vi "Actor Core.vi"(8 "error in":errorcluster, 11 "Nested in":refnum<class "Measurement GEN.lvclass">) -> (0 "error out":errorcluster, 3 "Actor out":refnum<class "Actor.lvclass">)   [LabVIEW 2020, in "Measurement GEN.lvlib" / "Measurement GEN.lvclass"]
doc: "(<B>Filename</B>: Actor Framework.lvlib:Actor.lvclass:Actor Core.vi)\n\nReceives messages to the actor, reacts to them, and initiates any error handling that may shut the actor down.\n\nDescendant classes may override this VI to append parallel tasks for the actor to complete while it handles messages. Overrides use the Call Parent Method node."
uses:
  Measurement GEN.lvclass
  <vilib>/ActorFramework/Stop Msg/Stop Msg.lvclass
  <vilib>/ActorFramework/Actor/Actor.lvclass
  F Generator Messages/Graficar datos Msg/Graficar datos Msg.lvclass
  <vilib>/measure/NI_MABase.lvlib
  C:/Program Files/National Instruments/LabVIEW 2020/vi.lib/ActorFramework/Actor/Actor.lvclass
  C:/Users/deLili/Desktop/UDLSB IET/701/Instrumentacion Virtual/Fork/AF-CML-TAREA/AF-CML-Tarea/Measurement GEN/Measurement GEN.lvclass
types:
  T1 = cluster{"Frecuencia":refnum<user-event>, "Amplitud":refnum<user-event>, "Stop":refnum<user-event>, "Start/Stop HL":refnum<user-event>, "Tipo Señal":refnum<user-event>}
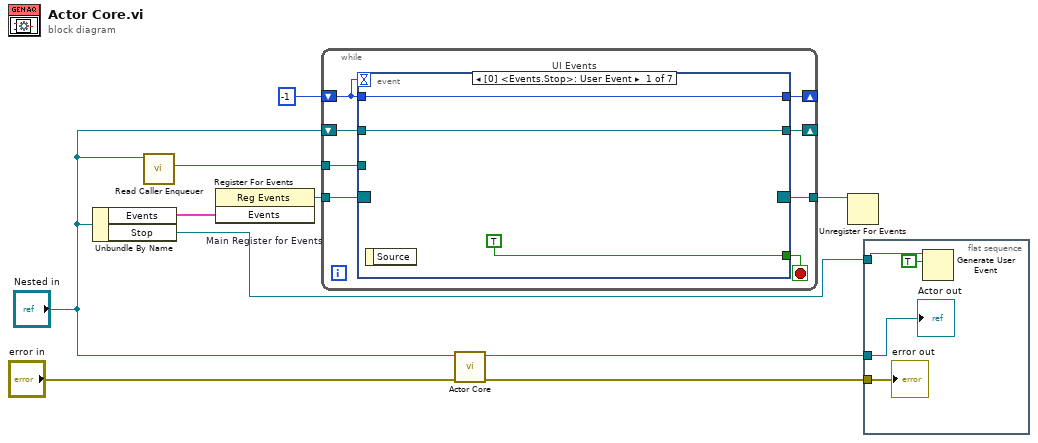
[diagram p0: block diagram]
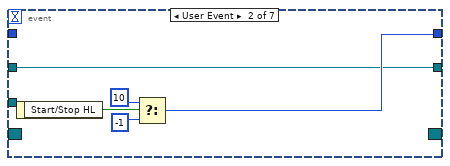
[diagram p2: hidden frame]
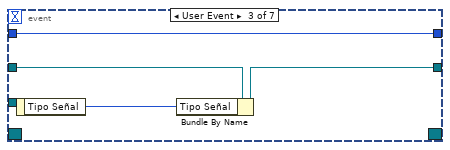
[diagram p3: hidden frame]
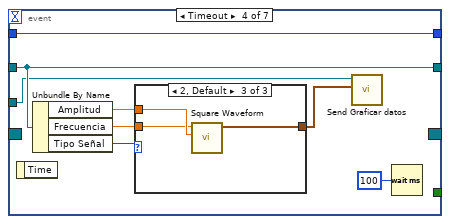
[diagram p4: hidden frame]
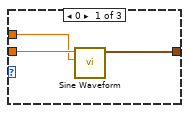
[diagram p5: hidden frame]
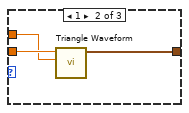
[diagram p6: hidden frame]
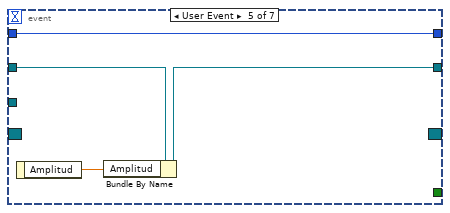
[diagram p7: hidden frame]
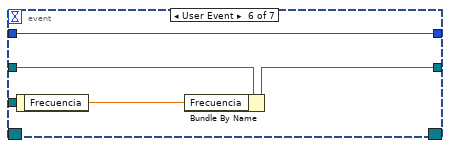
[diagram p8: hidden frame]
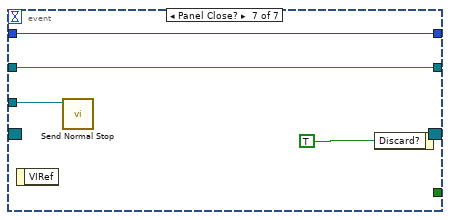
[diagram p9: hidden frame]
diagram:
  n1 = Unbundle By Name("Nested in") -> ("Events"=w7:T1, "Stop"=w4:refnum<user-event>)
  n2 = call <vilib>:"Read Caller Enqueuer.vi"("Actor"="Nested in") -> ("Caller Enqueuer"=w1:refnum<class "Message Enqueuer.lvclass">)  [unwired: 10 in]
  n3 = register-events "Main Register for Events"(w7) -> (reference out=w8:refnum<event-registration>)  [unwired: 2 in, 1 out]
  n4 = while {
    tunnel: w8 -> [w11]
    tunnel: [w17] -> w6
    shift-right: [w14] -> _
    shift-left: -1 -> [w15]
    shift-right: [w13] -> _
    shift-left: "Nested in" -> [w16]
    tunnel: w1 -> [w12]
    stop <- w18 stop-if-true
    n5 = event "UI Events" shown="[0] <Events.Stop>: User Event" {
      selector: w11 -> [_ _ _ _ _ _ _]
      dyn-events: [_ _ _ _ _ _ _] -> w17
      timeout: w15 -> [_ _ _ _ _ _ _]
      tunnel: [TRUE _ _ _ _ _ _] -> w18
      tunnel: w16 -> [w20 w22 w29 w37 w50 w55 w57]
      tunnel: w15 -> [w19 _ w30 w38 w51 w54 w58]
      tunnel: [w19 w23 w30 w38 w51 w54 w58] -> w14
      tunnel: [w20 w22 w28 w37 w49 w53 w57] -> w13
      tunnel: w12 -> [_ _ _ w36 _ _ w56]
      event User Event {
        n6 = event-data() -> ()  [unwired: 1 in, 1 out]
      }
      event User Event {
        n7 = event-data() -> ("Start/Stop HL"=w26:bool)  [unwired: 1 in]
        n8 = Select(t=10, s=w26, f=-1) -> (s? t:f=w23:i32)
      }
      event User Event {
        n9 = event-data() -> ("Tipo Señal"=w27:u16)  [unwired: 1 in]
        n10 = Bundle By Name(cluster=w29, "Tipo Señal"=w27) -> (w28:refnum<class "Measurement GEN.lvclass">)
      }
      event Timeout {
        n11 = event-data() -> ()  [unwired: 1 in, 1 out]
        n12 = Unbundle By Name(w37) -> ("Amplitud"=w32:dbl, "Frecuencia"=w33:dbl, "Tipo Señal"=w34:u16)
        n13 = case shown="2, Default" w34 {
          tunnel: w33 -> [w41 w44 w46]
          tunnel: w32 -> [w40 w43 w47]
          tunnel: [w39 w42 w45] -> w31
          frame 0 {
            n14 = call <vilib>:"Sine Waveform.vi"("amplitude"=w40, "frequency"=w41) -> ("signal out"=w39:waveform(dbl))  [unwired: 8 in, 1 out]
          }
          frame 1 {
            n15 = call <vilib>:"Triangle Waveform.vi"("amplitude"=w43, "frequency"=w44) -> ("signal out"=w42:waveform(dbl))  [unwired: 8 in, 1 out]
          }
          frame 2, Default {
            n16 = call <vilib>:"Square Waveform.vi"("amplitude"=w47, "frequency"=w46) -> ("signal out"=w45:waveform(dbl))  [unwired: 8 in, 1 out]
          }
        }
        n17 = call "Send Graficar datos.vi"("signal out"=w31, "Message Enqueuer"=w36) -> ()  [unwired: 8 in, 2 out]
        n18 = Wait (ms)(milliseconds to wait=u32 100) -> ()  [unwired: 1 out]
      }
      event User Event {
        n19 = event-data() -> ("Amplitud"=w48:dbl)  [unwired: 1 in]
        n20 = Bundle By Name(cluster=w50, "Amplitud"=w48) -> (w49:refnum<class "Measurement GEN.lvclass">)
      }
      event User Event {
        n21 = event-data() -> ("Frecuencia"=w52:dbl)  [unwired: 1 in]
        n22 = Bundle By Name(cluster=w55, "Frecuencia"=w52) -> (w53:refnum<class "Measurement GEN.lvclass">)
      }
      event Panel Close? {
        n23 = event-data() -> ()  [unwired: 1 in, 1 out]
        n24 = call <vilib>:"Send Normal Stop.vi"("Message Enqueuer"=w56) -> ()  [unwired: 10 in, 1 out]
        n25 = event-data("Discard?"=TRUE) -> ()  [unwired: 1 in, 1 out]
      }
    }
  }
  n26 = call-parent "Actor Core.vi"("error in"="error in", "Actor in"="Nested in") -> ("error out"=w10:errorcluster, "Actor out"=w9:refnum<class "Actor.lvclass">)  [unwired: 8 in]
  n27 = Unregister For Events(event registration refnum=w6) -> ()  [unwired: 1 in, 1 out]
  n28 = flat-sequence {
    tunnel: w10 -> [w63]
    tunnel: w9 -> [w62]
    tunnel: w4 -> [w60]
    frame #0 {
      n29 = Generate User Event(user event=w60, event data cluster=TRUE) -> ()  [unwired: 2 in, 2 out]
      "error out" <- w63
      "Actor out" <- w62
    }
  }
